vi "Bini output cluster ArchiveAndFtp.vi"(0 "Settings To Bini":T1={"Site ID"="", "File Management cluster"={"Comp File Size"=FALSE, "File Handle Method"=enum."Archive and zip in place from file *.ext list", "file extention list"=[]}, "time stamp"=timestamp(0 s since 1904-01-01), "File output directories"={"Archive Location"=path "", "Archive Location 2"=path "<Not A Path>", "OutPut Path"=path "", "Directory(s) To Scan Files"=[]}, "Auto FTP"=FALSE, "Auto Archive"=FALSE, "FTP CRED Cluster"={"Host"="", "UserName"="", "PassWord"="", "FTP File Path"="", "Timeout (S)"=60, "ActivePasive"=FALSE, "Binary Ascii"=FALSE, "Remote Port"=21}, "hours old date mod(hours)"=2, "Email Notification Cluster"={"Mail Server"="", "Return Address"="", "Email User Name"="", "Password"=""}, "Email Recipiant List"=[], "Addresses to Ping"=[]} {"FTP CRED Cluster"."Timeout (S)" min=0 max=300 step=1}) -> (15 "Bini Error out":errorcluster)   [LabVIEW 2011]
uses:
  Bini ArchiveAndFtpCluster.ctl
  Controls/File Management.ctl
  Controls/File Path directories.ctl
  Controls/FTP Credintials.ctl
  Controls/Ping address and email notify.ctl
  Controls/PingElements.ctl
panel:
  # "File Handling Method"
  # "Passive"
  # "Active"
  # "Binary"
  # "Ascii"
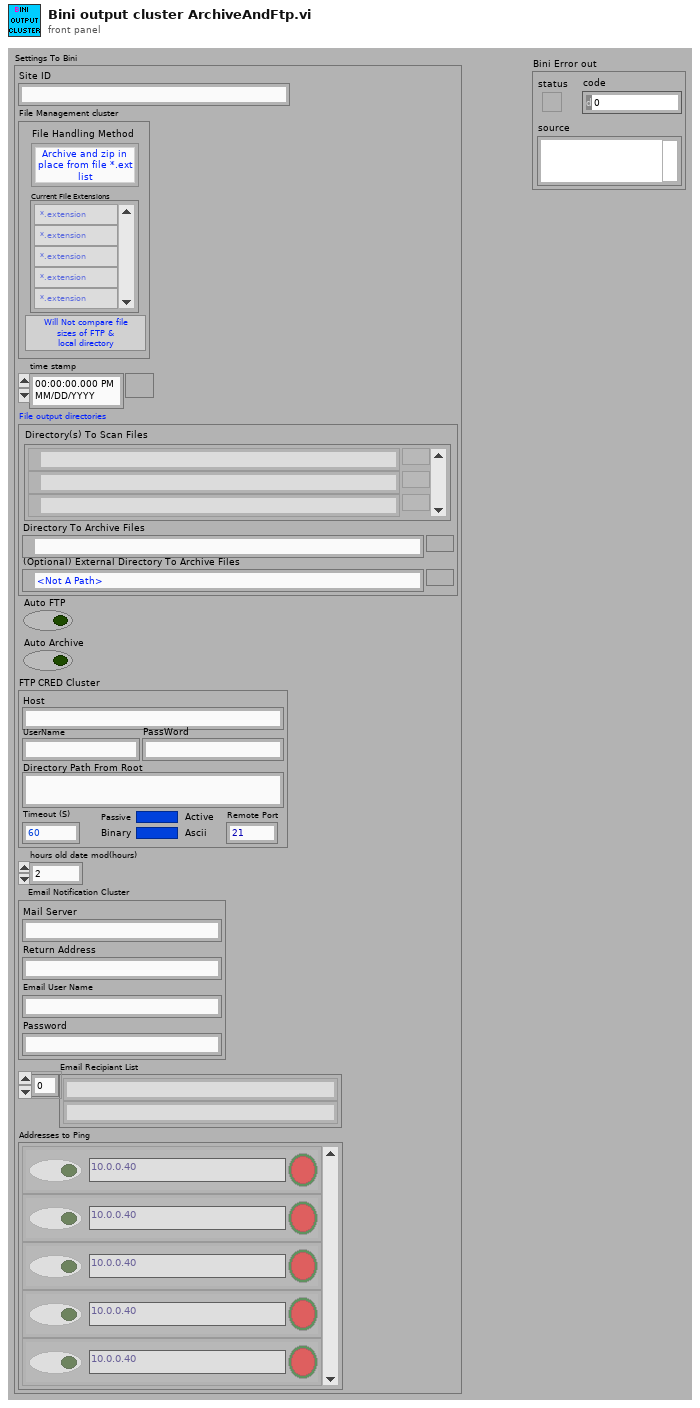
[diagram p1: front panel]
types:
  T1 = typedef "Bini ArchiveAndFtpCluster.ctl" = cluster{"Site ID":string, "File Management cluster":T2, "time stamp":timestamp, "File output directories":T3, "Auto FTP":bool, "Auto Archive":bool, "FTP CRED Cluster":T4, "hours old date mod(hours)":u8, "Email Notification Cluster":T5, "Email Recipiant List":string[], "Addresses to Ping":T6}
  T2 = typedef "File Management.ctl" = cluster{"Comp File Size":bool, "File Handle Method":enum16{"Archive and zip in place from file *.ext list", "Archive and zip ALL file Types to archive directory", "Archive and zip to archive directory from file *.ext list", "Perform no file management"}, "file extention list":string[]}
  T3 = typedef "File Path directories.ctl" = cluster{"Archive Location":path, "Archive Location 2":path, "OutPut Path":path, "Directory(s) To Scan Files":path[]}
  T4 = typedef "FTP Credintials.ctl" = cluster{"Host":string, "UserName":string, "PassWord":string, "FTP File Path":string, "Timeout (S)":i32, "ActivePasive":bool, "Binary Ascii":bool, "Remote Port":u16}
  T5 = typedef "Ping address and email notify.ctl" = cluster{"Mail Server":string, "Return Address":string, "Email User Name":string, "Password":string}
  T6 = typedef "PingElements.ctl" = cluster{"AddressNode 1":string, "Response 1":bool, "Ping on Address 1":bool}[]
  T7 = enum16{"open", "replace", "create", "open or create", "replace or create", "replace or create with confirmation"}
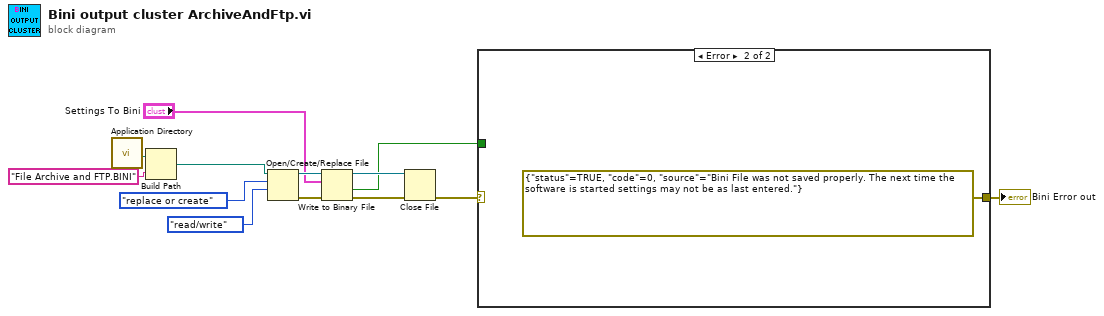
[diagram p0: block diagram]
diagram:
  n1 = call <vilib>:"Application Directory.vi"() -> ("Application Directory"=w3:path)
  n2 = Build Path(base path=w3, name or relative path="File Archive and FTP.BINI") -> (appended path=w7:path)
  n3 = Open/Create/Replace File(file path (use dialog)=w7, operation (0:open)=T7."replace or create", access (0:read/write)=enum16{"read/write", "read-only", "write-only"}."read/write") -> (refnum out=w6:refnum<file>, error out=w5:errorcluster)  [unwired: 3 in, 1 out]
  n4 = Write to Binary File(file (use dialog)=w6, data="Settings To Bini", error in=w5) -> (refnum out=w10:refnum<file>, cancelled=w4:bool, error out=w11:errorcluster)  [unwired: 3 in]
  n5 = Close File(refnum=w10, error in=w11) -> (error out=w12:errorcluster)  [unwired: 1 out]
  n6 = case shown="Error" w12 {
    selector: w12 -> [w14 _]
    tunnel: w4 -> [_ _]
    tunnel: [w14 errorcluster {"status"=TRUE, "code"=0, "source"="Bini File was not saved properly. The next time the software is started settings may not be as last entered."} ("error IO")] -> w13
    frame No Error {
    }
    frame Error {
    }
  }
  "Bini Error out" <- w13
